vi "Test PC.vi"() -> ()   [LabVIEW 2018]
uses:
  cRIO RT/FPGA Bitfile Register Operations/Scalar IO Operations/TypeDefs/Cluster Configuration.ctl
  <vilib>/Utility/Data Type/Type Definitions/Data Type.ctl
  cRIO RT/TypeDefs/Simple cluster.ctl
  cRIO RT/FPGA Bitfile Register Operations/Scalar IO Operations/Scalar IO Operations.lvlib
  <vilib>/Utility/Data Type/NI_Data Type.lvlib
panel:
  out "Array of VData":variant[](array[variant])
  out "Cluster Elements":variant[](array[variant])
  out "Cluster Configuration":T1
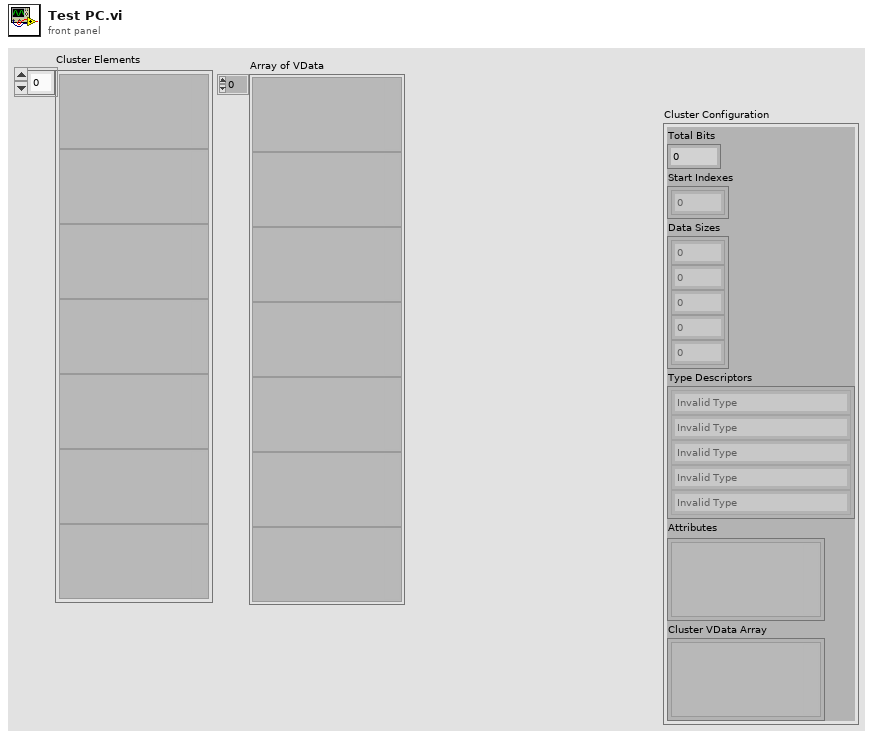
[diagram p1: front panel]
types:
  T1 = typedef "Scalar IO Operations.lvlib/Cluster Configuration.ctl" = cluster{"Total Bits":i32, "Start Indexes":i32[], "Data Sizes":i32[], "Type Descriptors":T2[], "Attributes":variant[], "Cluster VData Array":variant[]}
  T2 = typedef "NI_Data Type.lvlib/Data Type.ctl" = enum8{"Invalid Type", "Void", "I8", "I16", "I32", "I64", "U8", "U16", "U32", "U64", "Single Float", "Double Float", "Extended Float", "Single Complex", "Double Complex", "Extended Complex", "Enum U8", "Enum U16", "Enum U32", "Enum U64", "Single Float With Unit", "Double Float With Unit", "Extended Float With Unit", "Single Complex with Unit", "Double Complex with Unit", "Extended Complex with Unit", "Boolean", "String", "Path", "Picture", "Tag", "Array", "Cluster", "Variant", "LV Variant", "Waveform", "Timestamp", "Digital Waveform", "Digital Data", "ExpressData", "Refnum", "External Data", "VI", "Poly VI", "LabVIEW Class Instance", "Fixed Point"}
  T3 = typedef "Simple cluster.ctl" = cluster{"I16":i16, "U64":u64, "SGL":sgl, "Bool":bool, "FXP 12/6":fxp<+/-,12,6>}
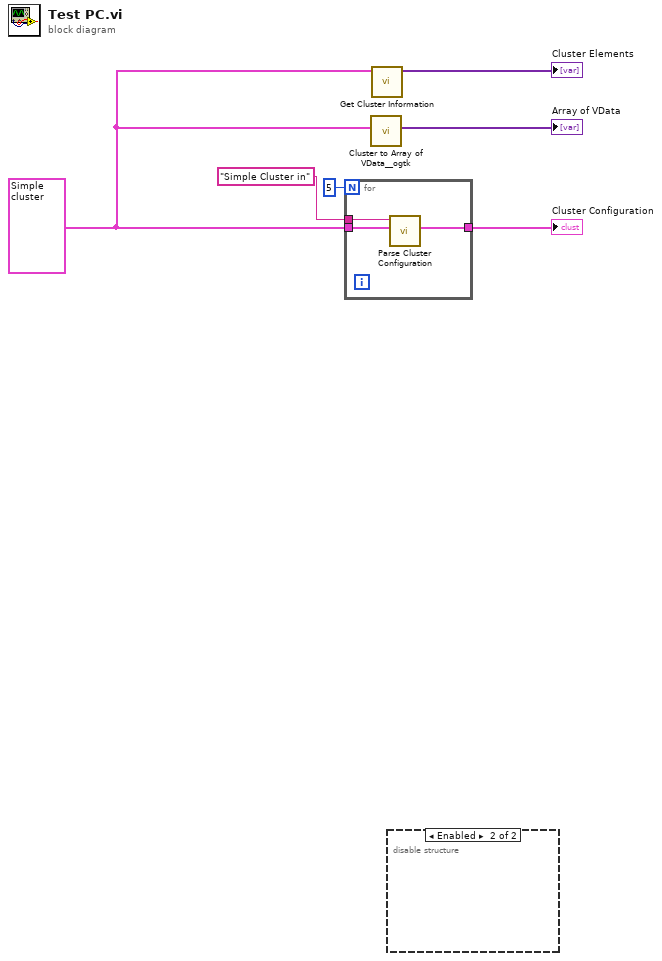
[diagram p0: block diagram]
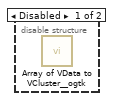
[diagram p2: hidden frame]
diagram:
  w2 = T3 {"I16"=123, "U64"=46456, "SGL"=0.65496, "Bool"=TRUE, "FXP 12/6"=0.0} ("Simple Cluster")
  n1 = for {
    N: 5 -> [_]
    tunnel: w2 -> [w9]
    tunnel: [w8] -> w6
    tunnel: "Simple Cluster in" ("Register Name in") -> [w7]
    n2 = call "Parse Cluster Configuration.vi"("Cluster in"=w9, "Register Name in"=w7) -> ("Cluster Configuration"=w8:T1)  [unwired: 8 in, 1 out]
  }
  "Cluster Configuration" <- w6
  n3 = call <userlib>:"Cluster to Array of VData__ogtk.vi"("Cluster"=w2) -> ("Array of VData"=→"Array of VData":variant[])  [unwired: 9 in, 1 out]
  n4 = call <vilib>:"Get Cluster Information.vi"("Variant"=w2) -> ("Cluster Elements"=→"Cluster Elements":variant[])  [unwired: 9 in, 1 out]
  n5 = disable-structure shown="Enabled" {
    frame Disabled {
      n6 = call <userlib>:"Array of VData to VCluster__ogtk.vi"() -> ()  [unwired: 10 in, 2 out]
    }
    frame Enabled {
    }
  }
